vi "Update Motor Setpoint Value.vi"(8 "error in (no error)":errorcluster, 9 "state mode":T1 items=["undefined", "angle", "velocity"], 10 "value":dbl, 11 "motor communication in":refnum<class "NI_Robotics_Motor Communication Ref.lvclass">) -> (0 "error out":errorcluster, 1 "failed?":bool, 3 "motor communication out":refnum<class "NI_Robotics_Motor Communication Ref.lvclass">)   [LabVIEW 2017, in "NI_Robotics_Motor Communication Ref.lvclass"]
uses:
  <vilib>/robotics/Actuation/Motor Communication Ref/NI_Robotics_Motor Communication Ref.lvclass
  <vilib>/robotics/Actuation/Motor Communication/Motor State Mode.ctl
  <vilib>/robotics/Actuation/Motor Communication Ref/NI_Robotics_Motor Communication Ref.lvclass/NI_Robotics_Motor Communication Ref.ctl
  <vilib>/robotics/Actuation/Motor Communication/Write to Motor State.vi
  <vilib>/robotics/Actuation/Motor Communication/NI_Robotics_Motor Communication.lvclass
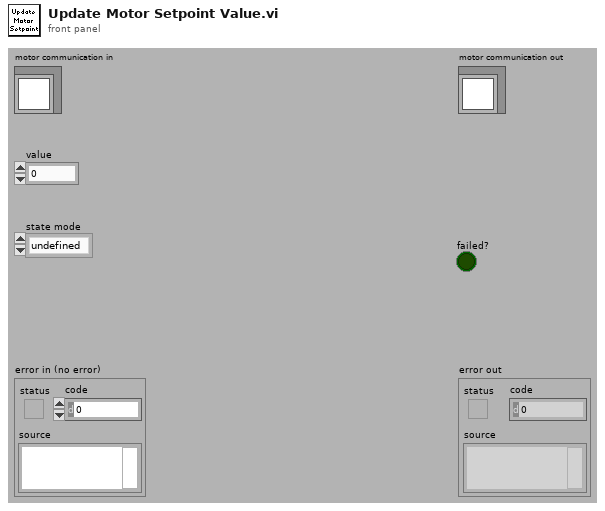
[diagram p1: front panel]
types:
  T1 = typedef "NI_Robotics_Motor Communication.lvclass/Motor State Mode.ctl" = u16
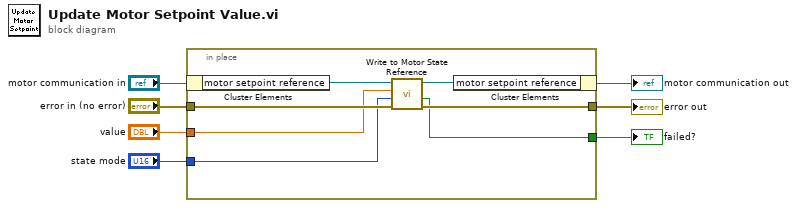
[diagram p0: block diagram]
diagram:
  n1 = in-place {
    in-place-border: "error in (no error)" -> [w12]
    in-place-border: "value" -> [w11]
    in-place-border: "state mode" -> [w10]
    in-place-border: [w9] -> w2
    in-place-border: [w8] -> w1
    n2 = in-place-cluster #1("motor communication in") -> ("motor setpoint reference"=w14:refnum<data-value>)
    n3 = call <vilib>:"Write to Motor State Reference.vi"("error in (no error)"=w12, "state mode"=w10, "value"=w11, "motor state ref in"=w14) -> ("error out"=w9:errorcluster, "failed?"=w8:bool, "motor state ref out"=w13:refnum<data-value>)  [unwired: 5 in]
    n4 = in-place-cluster #1("motor setpoint reference"=w13) -> (→"motor communication out":refnum<class "NI_Robotics_Motor Communication Ref.lvclass">)
  }
  "error out" <- w2
  "failed?" <- w1
